vi "RS485 Comm Test 1.vi"() -> ()   [LabVIEW 2014]
uses:
  ALPHA5 RS485/typedefs/Port Selection Info.ctl
  ALPHA5 RS485/ALPHA5 RS485.lvlib
panel:
  out "Check Result":bool
  out "Info Code 2":u16
  out "Info Data 2":u16
  out "FC":u8
  out "Amplifier Num":u8
  in  "Info Data":u16=65535 format="%.0x"
  in  "Info Code":u16 format="%.0x"
  out "error out":errorcluster
  in  "Port Selection Info":T1={"Port Name"="", "Amplifier Num"=1, "Baud Rate"=38400, "Char Formation"=enum."0"} {"Baud Rate" items=["38400"=38400, "19200"=19200, "9600"=9600, "115200"=0]; "Amplifier Num" max=31}
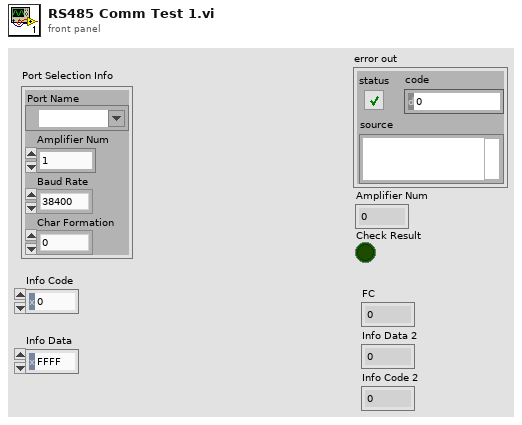
[diagram p1: front panel]
types:
  T1 = typedef "ALPHA5 RS485.lvlib/Port Selection Info.ctl" = cluster{"Port Name":refnum<visa-resource-name>, "Amplifier Num":u8, "Baud Rate":u32, "Char Formation":enum16{"0", "1", "2", "3", "4", "5"}}
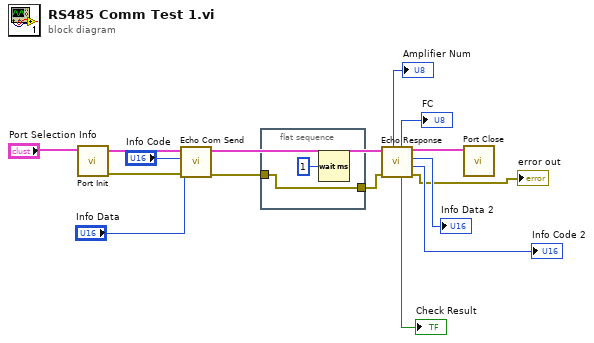
[diagram p0: block diagram]
diagram:
  n1 = call "Port Init.vi"("Port Selection Info In"="Port Selection Info") -> ("error out"=w13:errorcluster, "Port Selection Info Out"=w14:T1)  [unwired: 9 in]
  n2 = call "Echo Com Send.vi"("error in (no error)"=w13, "Info Data"="Info Data", "Info Code"="Info Code", "Port Selection Info"=w14) -> ("error out"=w2:errorcluster, "Port Selection Info Out"=w12:T1)  [unwired: 6 in]
  n3 = flat-sequence {
    tunnel: w2 -> [w16]
    tunnel: [w16] -> w1
    frame #0 {
      n4 = Wait (ms)(milliseconds to wait=u32 1) -> ()  [unwired: 1 out]
    }
  }
  n5 = call "Echo Response.vi"("error in (no error)"=w1, "Port Selection Info"=w12) -> ("error out"=→"error out":errorcluster, "Info Code"=→"Info Code 2":u16, "Info Data"=→"Info Data 2":u16, "Port Selection Info Out"=w3:T1, "Check Result"=→"Check Result":bool, "FC"=→"FC":u8, "Amplifier Num"=→"Amplifier Num":u8)  [unwired: 3 in]
  n6 = call "Port Close.vi"("Port Selection Info In"=w3) -> ()  [unwired: 10 in, 1 out]
